vi "Go2Angle.vi"(0 "VISA resource name":refnum<visa-resource-name>, 1 "Photodiode":refnum<visa-resource-name>, 5 "RotStage Det Angle Readout (°) 4":refnum<vi>, 6 "Excitation Power (uW) 2":refnum<vi>, 7 "Photodiode on?":bool, 9 "Axis ESP301 / RotStage":u16(ring) items=["LinStage"=1, "RotStage Detection"=2, "RotStage Excitation"=3], 11 "ESP301 Error":errorcluster, 12 "Photodiode error":errorcluster, 14 "Position (units)":dbl format="%.6g") -> (3 "Photodiode out":refnum<visa-resource-name>, 4 "VISA resource name out":refnum<visa-resource-name>, 10 "Photodiode":errorcluster, 15 "ESP301 Error out":errorcluster)   [LabVIEW 2019]
uses:
  Newport/Newport ESP301/Newport ESP301.lvlib
panel:
  out "Photodiode handle out":refnum<visa-resource-name> caption="instrument handle out"
  out "Excitation Power (uW)":dbl=0.2 caption="P    =" format="%#_3p"
  out "Motion Done":bool
  out "RotStage Det Angle Readout (°) 3":dbl=2.0 caption="Readout (°)" min=-360.0 max=360.0 format="%#_4g"
  out "RotStage Det Angle Readout (°)":dbl=2.0 caption="Readout (°)" min=-360.0 max=360.0 format="%#_4g"
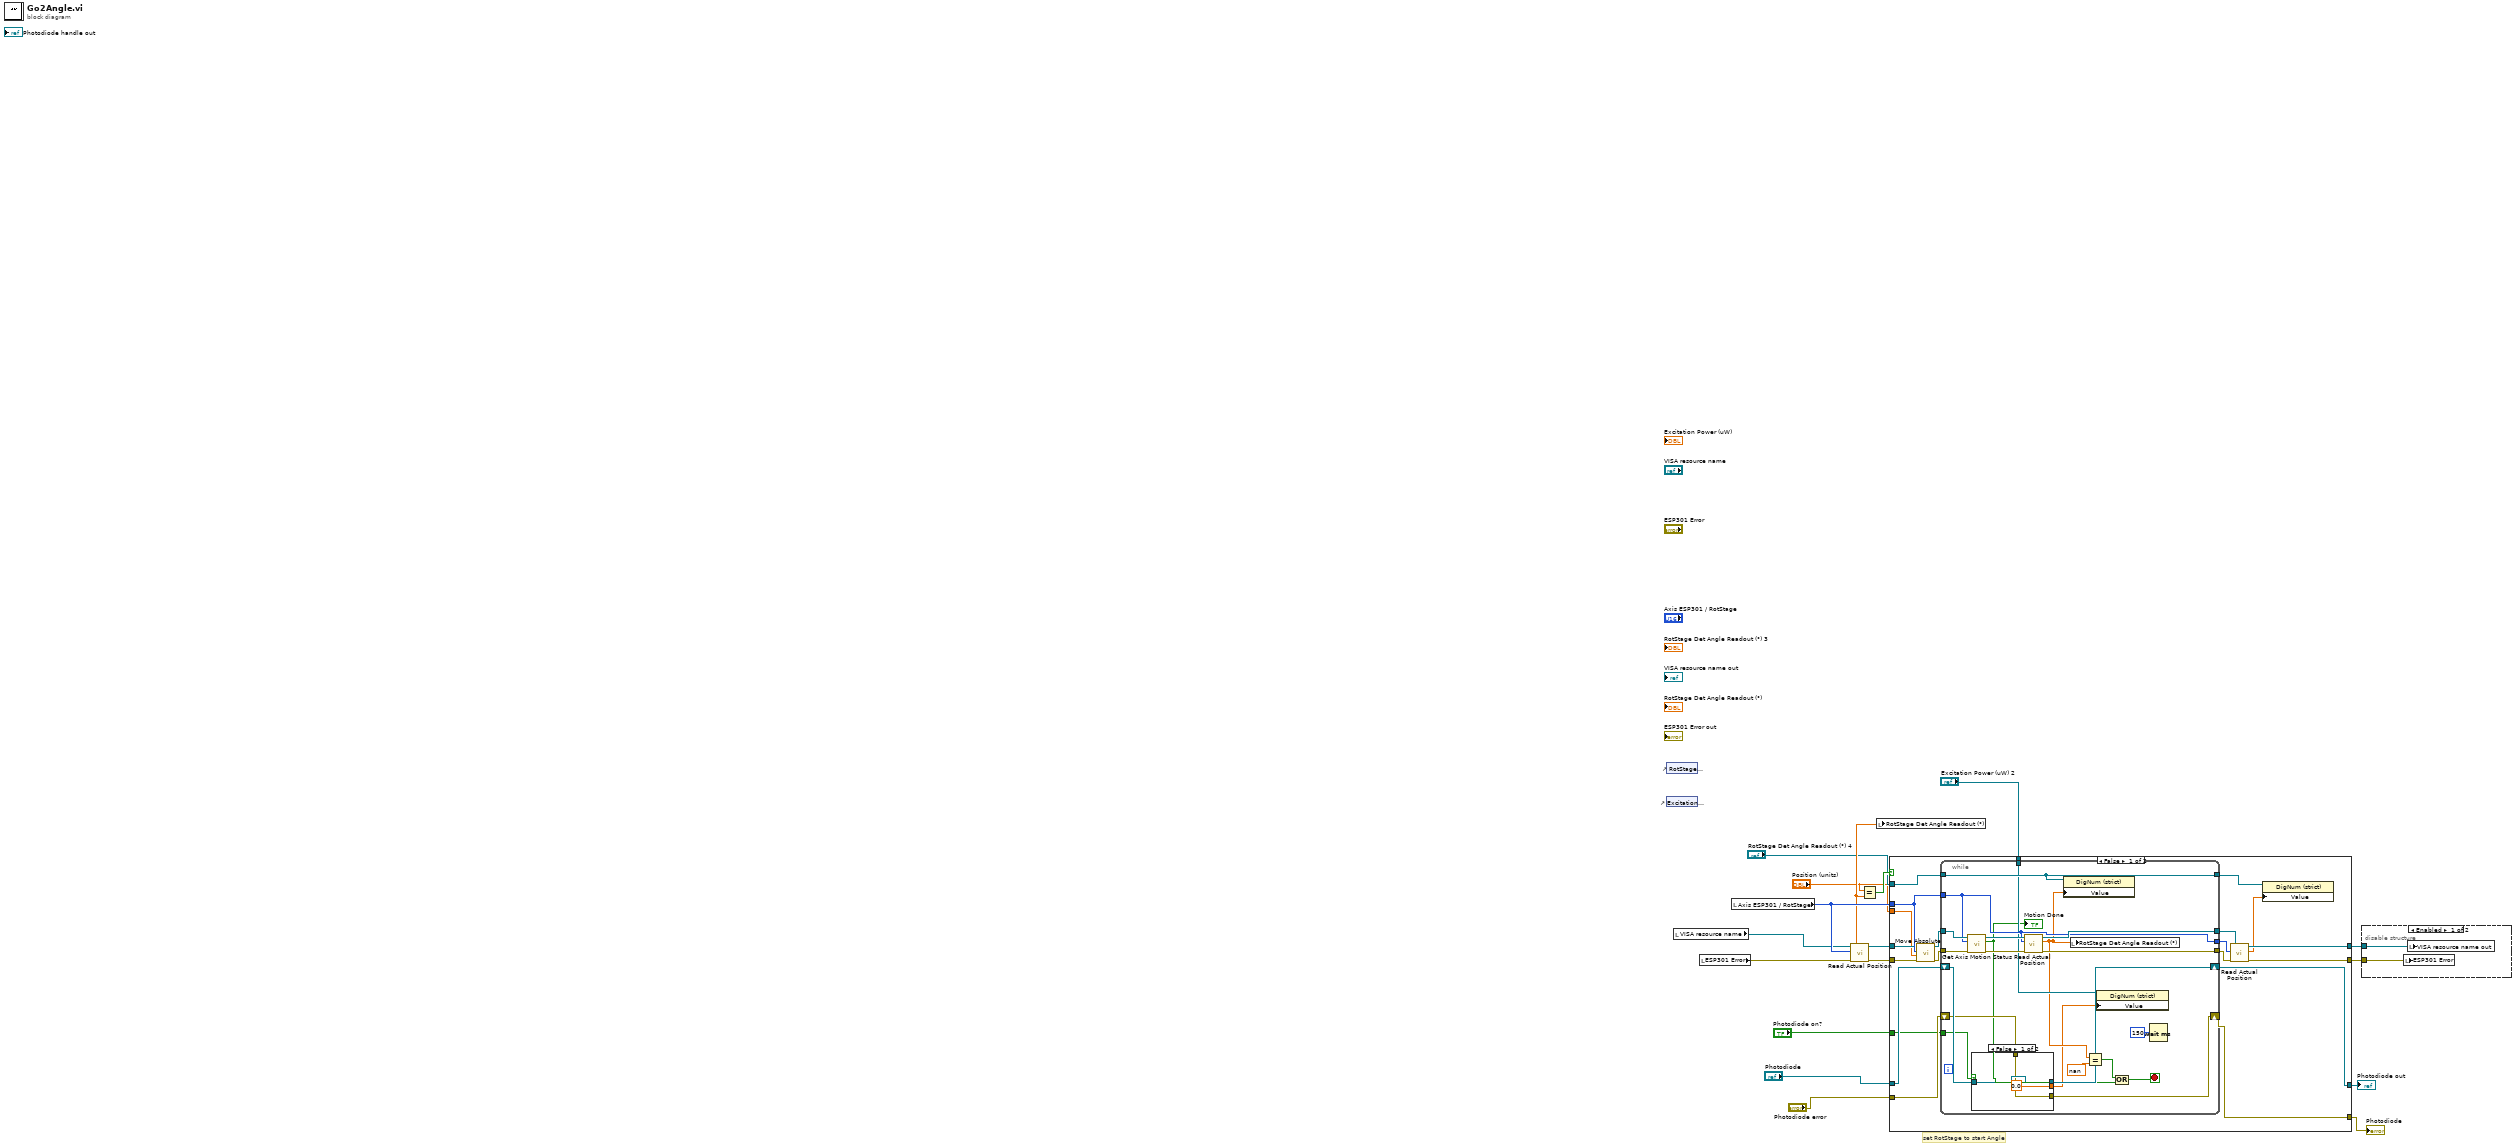
[diagram p0: block diagram]
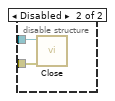
[diagram p2: hidden frame]
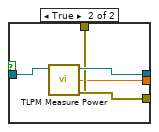
[diagram p3: hidden frame]
diagram:
  # "set RotStage to start Angle"
  n1 = control-ref of="RotStage Det Angle Readout (°)"() -> ()  [unwired: 1 out]
  n2 = control-ref of="Excitation Power (uW)"() -> ()  [unwired: 1 out]
  n3 = local read "VISA resource name"() -> (w3:refnum<visa-resource-name>)
  n4 = local read "ESP301 Error"() -> (w2:errorcluster)
  n5 = local read "Axis ESP301 / RotStage"() -> (w15:u16)
  n6 = call "Read Actual Position.vi"("error in (no error)"=w2, "Axis (1)"=w15, "VISA resource name"=w3) -> ("error out"=w13:errorcluster, "Position (units)"=w11:dbl, "VISA resource name out"=w12:refnum<visa-resource-name>)  [unwired: 2 in]
  n7 = Equal?(x="Position (units)", y=w11) -> (x = y?=w14:bool)
  n8 = local write "RotStage Det Angle Readout (°)"(w11) -> ()
  n9 = case shown="False" w14 {
    tunnel: [w28 w70] -> w17
    tunnel: [w29 w69] -> w16
    tunnel: w15 -> [w35 _]
    tunnel: w13 -> [w34 w69]
    tunnel: w12 -> [w33 w70]
    tunnel: "RotStage Det Angle Readout (°) 4" -> [w32 _]
    tunnel: "Position (units)" -> [w24 _]
    tunnel: "Photodiode" -> [w23 w68]
    tunnel: "Photodiode error" -> [w21 w67]
    tunnel: [w22 w68] -> w6
    tunnel: [w20 w67] -> w5
    tunnel: "Excitation Power (uW) 2" -> [w19 _]
    tunnel: "Photodiode on?" -> [w18 _]
    frame False {
      n10 = call "Move Absolute.vi"("error in (no error)"=w34, "Position (0 units)"=w24, "Axis (1)"=w35, "VISA resource name"=w33) -> ("error out"=w36:errorcluster, "VISA resource name out"=w37:refnum<visa-resource-name>)  [unwired: 2 in]
      n11 = while {
        tunnel: w35 -> [w52]
        tunnel: w32 -> [w51]
        tunnel: [w52] -> w27
        tunnel: [w51] -> w26
        shift-right: [w49] -> w22
        shift-left: w23 -> [w50]
        shift-right: [w40] -> w20
        shift-left: w21 -> [w48]
        tunnel: w19 -> [w47]
        tunnel: w18 -> [w39]
        tunnel: w37 -> [w58]
        tunnel: [w55] -> w31
        tunnel: w36 -> [w57]
        tunnel: [w53] -> w30
        stop <- w44 stop-if-true
        n12 = call "Get Axis Motion Status.vi"("error in (no error)"=w57, "Axis (1)"=w52, "VISA resource name"=w58) -> ("error out"=w54:errorcluster, "Motion Done"=w42:bool, "VISA resource name out"=w56:refnum<visa-resource-name>)  [unwired: 2 in]
        "Motion Done" <- w42
        n13 = case shown="False" w39 {
          tunnel: w50 -> [w61 w66]
          tunnel: [w61 w65] -> w49
          tunnel: w48 -> [w59 w63]
          tunnel: [0.0 w62] -> w41
          tunnel: [w59 w64] -> w40
          frame False {
          }
          frame True {
            n14 = call <instrlib>:"TLPM Measure Power.vi"("error in (no error)"=w63, "instrument handle"=w66) -> ("error out"=w64:errorcluster, "Power"=w62:dbl, "instrument handle out"=w65:refnum<visa-resource-name>)  [unwired: 7 in]
          }
        }
        n15 = call "Read Actual Position.vi"("error in (no error)"=w54, "Axis (1)"=w52, "VISA resource name"=w56) -> ("error out"=w53:errorcluster, "Position (units)"=w43:dbl, "VISA resource name out"=w55:refnum<visa-resource-name>)  [unwired: 2 in]
        n16 = property class="DigNum (strict)"(reference=w51, "Value"=w43) -> ()  [unwired: 1 in, 2 out]
        n17 = local write "RotStage Det Angle Readout (°)"(w43) -> ()
        n18 = Equal?(x=w43, y=nan) -> (x = y?=w45:bool)
        n19 = property class="DigNum (strict)"(reference=w47, "Value"=w41) -> ()  [unwired: 1 in, 2 out]
        n20 = Or(x=w45, y=w42) -> (x .or. y?=w44:bool)
        n21 = Wait (ms)(milliseconds to wait=u32 150) -> ()  [unwired: 1 out]
      }
      n22 = call "Read Actual Position.vi"("error in (no error)"=w30, "Axis (1)"=w27, "VISA resource name"=w31) -> ("error out"=w29:errorcluster, "Position (units)"=w25:dbl, "VISA resource name out"=w28:refnum<visa-resource-name>)  [unwired: 2 in]
      n23 = property class="DigNum (strict)"(reference=w26, "Value"=w25) -> ()  [unwired: 1 in, 2 out]
    }
    frame True {
    }
  }
  "Photodiode out" <- w6
  "Photodiode" <- w5
  n24 = disable-structure shown="Enabled" {
    disable-tunnel: w17 -> [w72 w74]
    disable-tunnel: w16 -> [w71 w73]
    frame Enabled {
      n25 = local write "ESP301 Error"(w71) -> ()
      n26 = local write "VISA resource name out"(w72) -> ()
    }
    frame Disabled {
      n27 = call "Close.vi"("error in (no error)"=w73, "VISA resource name"=w74) -> ()  [unwired: 9 in, 1 out]
    }
  }
